vi "CNTRLR - State Change.vi"(8 "error in (no error)":errorcluster, 11 "View Model":T1) -> (0 "error out":errorcluster, 3 "View Model":T1)   [LabVIEW 2017]
doc: "This SubVI check IF Current State = Next State THEN do nothing, because\nthis step will be processing in State Proc.vi ELSE do actions for transition\nbetween steps OR/AND set up Next Step as Current Step for further processing"
uses:
  View Model/Controls/View Model.ctl
  View Model/Controls/Shared Model.ctl
  Error Handler/Controls/Error Model.ctl
  Error Handler/Controls/Error Message.ctl
  Error Handler/Controls/Error Level.ctl
  Configuration/Controls/Database Model.ctl
  Configuration/Controls/Database Message.ctl
  Configuration/Controls/Database Command.ctl
  Configuration/Controls/Database Overhead.ctl
  Configuration/Controls/Database Status.ctl
  Configuration/Controls/Database Record.ctl
  Configuration/Controls/Database - Rule Record.ctl
  Controls/CNTRLR - Wash Step.ctl
  Controls/CNTRLR - Position.ctl
  Controls/CNTRLR - Model.ctl
  Controls/CNTRLR - Message.ctl
  Controls/CNTRLR - Command.ctl
  Controls/CNTRLR - Overhead.ctl
  Controls/CNTRLR - State.ctl
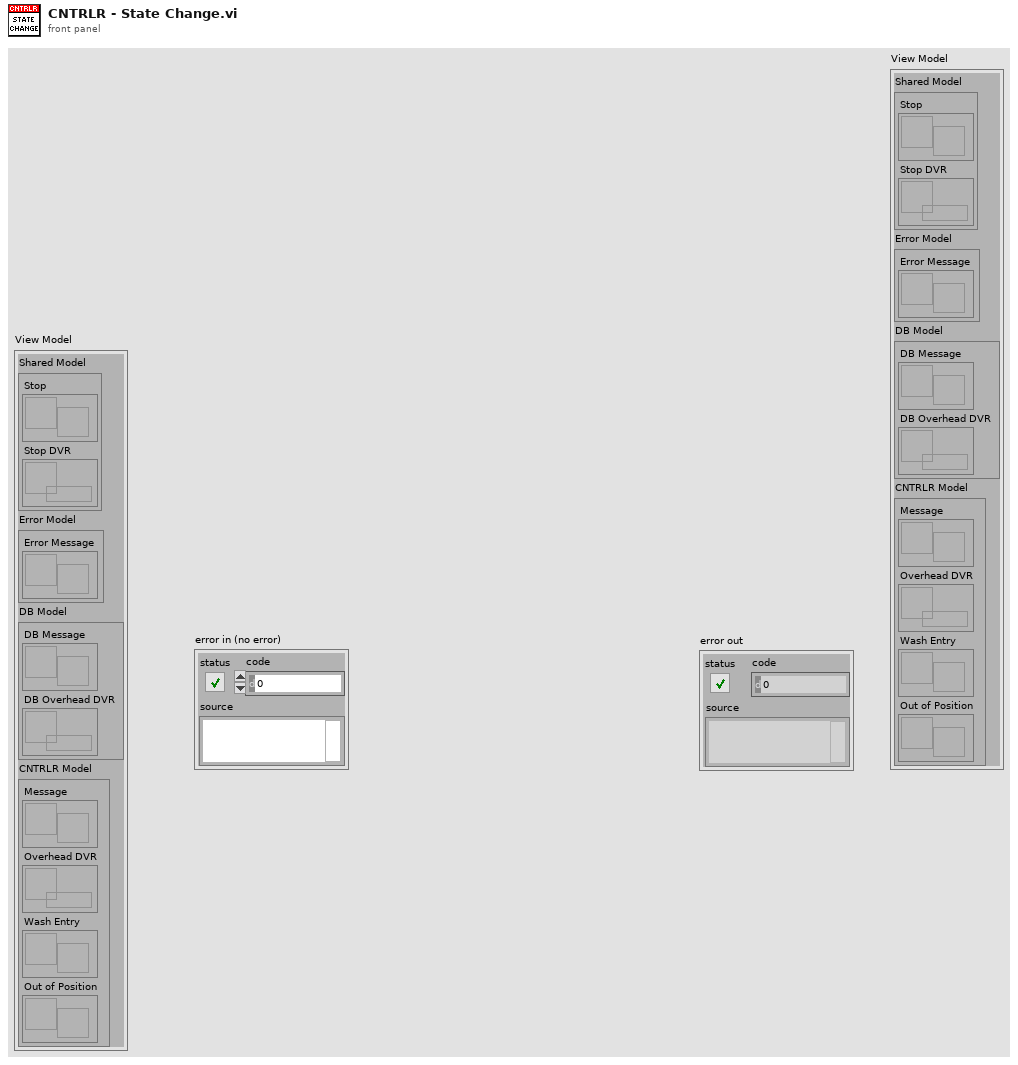
[diagram p1: front panel]
types:
  T1 = typedef "View Model.ctl" = cluster{"Shared Model":T2, "Error Model":T3, "DB Model":T4, "CNTRLR Model":T5}
  T2 = typedef "Shared Model.ctl" = cluster{"Stop":refnum<user-event>, "Stop DVR":refnum<data-value>}
  T3 = typedef "Error Model.ctl" = cluster{"Error Message":refnum<user-event>}
  T4 = typedef "Database Model.ctl" = cluster{"DB Message":refnum<user-event>, "DB Overhead DVR":refnum<data-value>}
  T5 = typedef "CNTRLR - Model.ctl" = cluster{"Message":refnum<user-event>, "Overhead DVR":refnum<data-value>, "Wash Entry":refnum<user-event>, "Out of Position":refnum<user-event>}
  T6 = typedef "CNTRLR - State.ctl" = enum16{"Initial", "Wait for Start", "Start State", "Wait for Vehicle Position", "Wash Step Execution", "Wash Step/Cycle Complete", "Wash Exit", "Wash Abort/Terminate"}
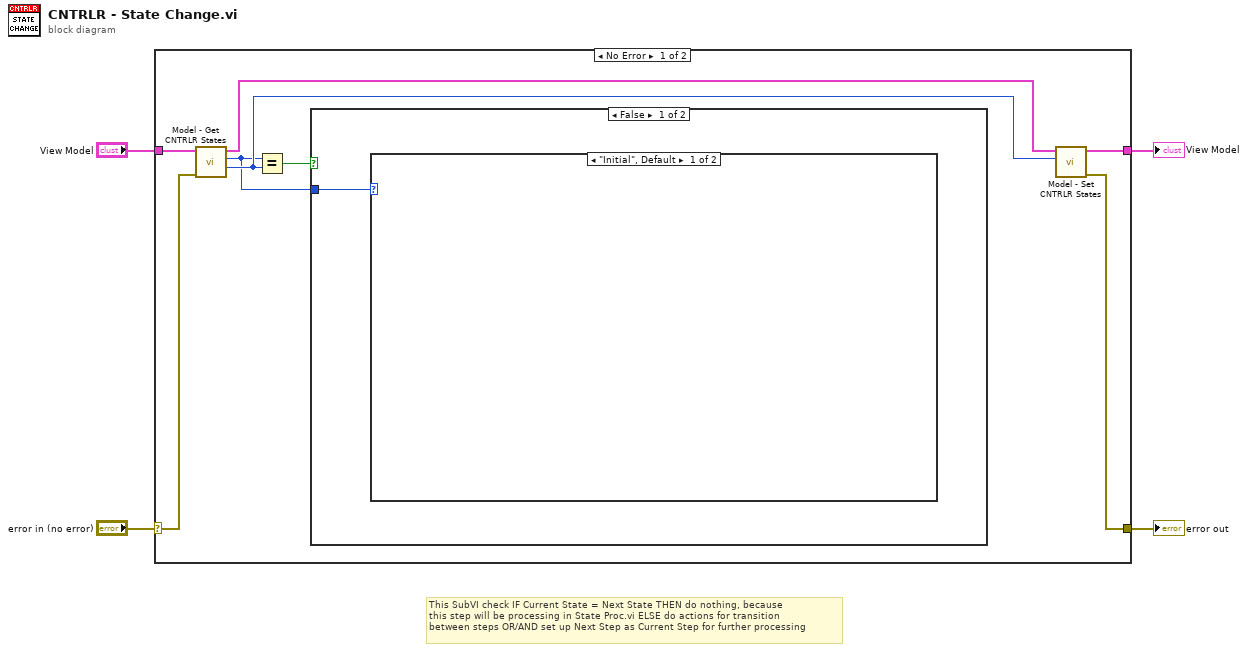
[diagram p0: block diagram]
diagram:
  # "This SubVI check IF Current State = Next State THEN do nothing, because\nthis step will be processing in State Proc.vi ELSE do actions for transition\nbetween steps OR/AND set up Next Step as Current Step for further processing"
  n1 = case shown="No Error" "error in (no error)" {
    selector: "error in (no error)" -> [w12 w15]
    tunnel: [w8 w15] -> w3
    tunnel: "View Model" -> [w11 w14]
    tunnel: [w9 w14] -> w1
    frame No Error {
      n2 = call "Model - Get CNTRLR States.vi"("error in (no error)"=w12, "View Model"=w11) -> ("Next State"=w6:T6, "Current State"=w5:T6, "View Model"=w10:T1)  [unwired: 6 in, 1 out]
      n3 = Equal?(x=w5, y=w6) -> (x = y?=w7:bool)
      n4 = case shown="False" w7 {
        tunnel: w5 -> [w13 _]
        frame False {
          n5 = case shown="\"Initial\", Default" w13 {
            frame "Initial", Default {
            }
            frame "Wait for Start" {
            }
          }
        }
        frame True {
        }
      }
      n6 = call "Model - Set CNTRLR States.vi"("Current State"=w6, "View Model"=w10) -> ("error out"=w8:errorcluster, "View Model"=w9:T1)  [unwired: 8 in]
    }
    frame Error {
    }
  }
  "error out" <- w3
  "View Model" <- w1
